vi "simplePID Memory Read_FXP.vi"(1 "channel (0)":u16, 3 "Input Selector":u16) -> (4 "Memory Out":refnum<k21>="Data", 15 "state out":T1)   [LabVIEW 2020]
uses:
  Typedef/niFpgaPID_PIDState_FXP.ctl
  <vilib>/rvi/Memory/Memory_Emulation/nirvimemoryEmulation.vi
  <vilib>/rvi/Memory/Memory_Emulation/nirvimemoryFastEmulation.vi
  <vilib>/rvi/DataTransferAndStorage/Container/Common/niFpgaContainerGetUniqueNameForEmu.vi
  <vilib>/rvi/Memory/Memory_Emulation/niFpgaMemoryEmulationCacheClearOnFirstRun.vi
  <vilib>/rvi/Memory/Memory_Emulation/nirvimemoryEmulationManagerCache_MakeExclusive.vi
  <vilib>/rvi/Memory/Memory_Emulation/niFpgaMemoryEmulationValidateCache.vi
  <vilib>/rvi/Memory/Memory_Emulation/nirvimemoryEmulationManagerCache_InsertValue.vi
  <vilib>/Utility/error.llb/Clear Errors.vi
  <vilib>/rvi/Memory/Memory_Emulation/nirvimemoryEmulationManagerCache_ReleaseExclusive.vi
  <vilib>/rvi/Memory/Memory_Emulation/nirvimemoryEmulationManagerCache_GetValue.vi
  <vilib>/rvi/Emulation/niFpgaEmulationIsFPGAContextNoSignature.vi
  <vilib>/rvi/Emulation/niFpgaSctlEmulationGetInTimedLoop.vi
  <vilib>/rvi/Memory/Memory_Emulation/nirvimemoryEmulationManagerCache_SetValue.vi
  <vilib>/rvi/Emulation/niFpgaSctlEmulationResourceMgr.vi
  <vilib>/rvi/DataTransferAndStorage/Container/XNode/niFpgaContainer.xnode
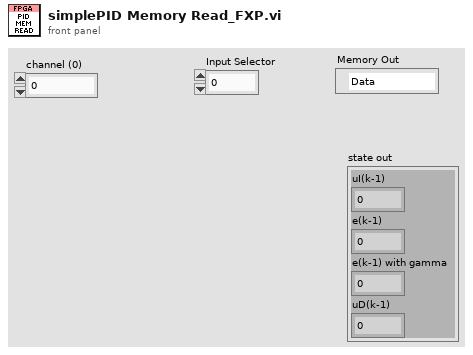
[diagram p1: front panel]
types:
  T1 = typedef "niFpgaPID_PIDState_FXP.ctl" = cluster{"uI(k-1)":fxp<+/-,20,12>, "e(k-1)":fxp<+/-,16,10>, "e(k-1) with gamma":fxp<+/-,16,10>, "uD(k-1)":fxp<+/-,20,12>}
  T2 = cluster{"data 1":fxp<+/-,20,12>, "data 2":fxp<+/-,16,10>, "data 3":fxp<+/-,16,10>, "data 4":fxp<+/-,20,12>}
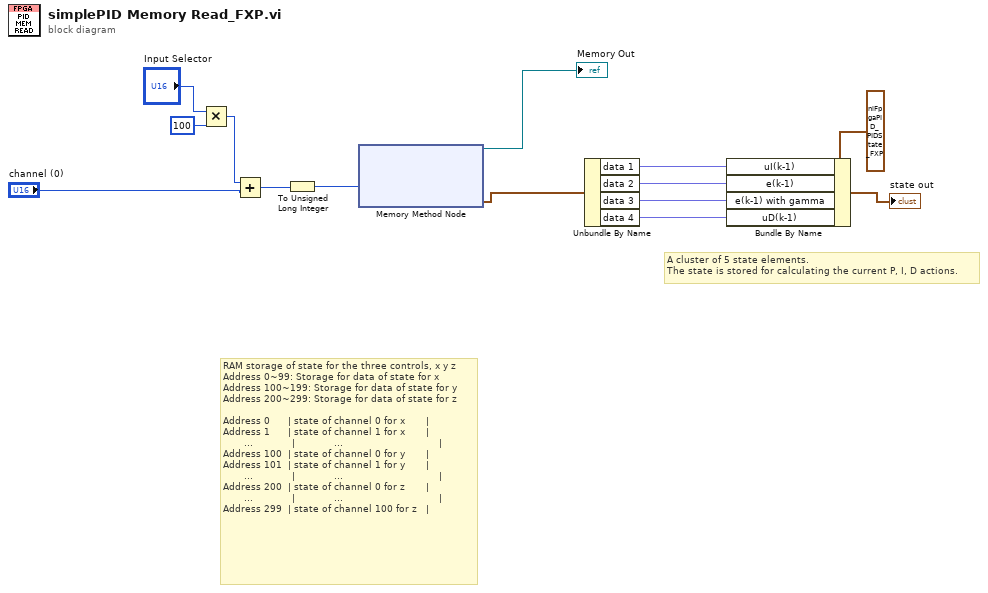
[diagram p0: block diagram]
diagram:
  # "RAM storage of state for the three controls, x y z\nAddress 0~99: Storage for data of state for x\nAddress 100~199: Storage for data of state for y\nAddress 200~299: Storage for data of state for z \n                                                                        \nAddress 0      | state of channel 0 for x       | \nAddress 1      | state of channel 1 for x       | \n       ...             |             ...                                |\nAddress 100  | state of channel 0 for y       | \nAddress 101  | state of channel 1 for y       | \n       ...             |             ...                                |\nAddress 200  | state of channel 0 for z       | \n       ...             |             ...                                |\nAddress 299  | state of channel 100 for z   |"
  # "A cluster of 5 state elements.\nThe state is stored for calculating the current P, I, D actions."
  n1 = Multiply(x="Input Selector", y=u16 100) -> (x*y=w7:u16)
  n2 = Add(x=w7, y="channel (0)") -> (x+y=w5:u16)
  n3 = To Unsigned Long Integer(number=w5) -> (unsigned 32bit integer=w3:u32)
  n4 = xnode ("Memory Method Node")("Address"=w3) -> ("Data"=w2:T2, "Memory Out"=→"Memory Out":refnum<k21>)  [unwired: 1 in]
  n5 = Unbundle By Name(w2) -> ("data 1"=w9:fxp<+/-,20,12>, "data 2"=w10:fxp<+/-,16,10>, "data 3"=w11:fxp<+/-,16,10>, "data 4"=w12:fxp<+/-,20,12>)
  n6 = Bundle By Name(cluster=T1 {"uI(k-1)"=0.0, "e(k-1)"=0.0, "e(k-1) with gamma"=0.0, "uD(k-1)"=0.0} ("state out"), "uI(k-1)"=w9, "e(k-1)"=w10, "e(k-1) with gamma"=w11, "uD(k-1)"=w12) -> (→"state out":T1)
